vi "Add Injector.vi"(7 "Max Shots":T1(ring)=enum."1", 8 "error in (no error)":errorcluster, 9 "Stages":string[](array[string])=["Boost", "Battery", "Off"], 10 "Controls":T3[](array[typedef]) {"Data Type" format="%.0x"}, 11 "Item Ref":T2=18446744073709551615 format="%.0x") -> (0 "error out":errorcluster, 3 "Item Ref out":T2=18446744073709551615 format="%.0x")   [LabVIEW 2015, in "Fuel Injector Analysis Addon System Explorer.lvlib"]
uses:
  Fuel Injector Analysis Addon System Explorer.lvlib
  <vilib>/NI Veristand/Custom Device API/Custom Device Item Ref.ctl
  Shared/Types/Register.Info.ctl
  Shared/Types/FPGA Data Types.ctl
  FPGA/Injection Capture IP/Types/Injection.Global.Settings.ctl
  Shared/Constants.vi
  <vilib>/NI Veristand/Custom Device API/Set Item Property (Variant).vi
  <vilib>/NI Veristand/Custom Device Tools/Custom Device Utility Library/NI VeriStand - Search for Item by GUID.vi
  <vilib>/NI Veristand/Custom Device Tools/Custom Device Utility Library/NI VeriStand - Search for All Items by GUID.vi
  Shared/Fuel Injector Analysis Addon Shared.lvlib
  <vilib>/NI Veristand/Custom Device API/Custom Device API.lvlib
  <vilib>/NI Veristand/Custom Device Tools/Custom Device Utility Library/Custom Device Utility Library.lvlib
panel:
  in  "Tags":string
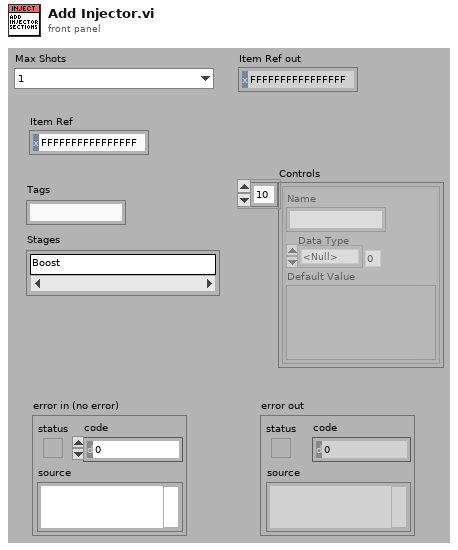
[diagram p1: front panel]
types:
  T1 = enum16{"0", "1", "2", "3", "4", "5", "6", "7", "8"}
  T2 = typedef "Custom Device API.lvlib/Custom Device Item Ref.ctl" = u64
  T3 = typedef "Fuel Injector Analysis Addon Shared.lvlib/Register.Info.ctl" = cluster{"Name":string, "Data Type":T4, "Default Value":variant}
  T4 = typedef "Fuel Injector Analysis Addon Shared.lvlib/FPGA Data Types.ctl" = enum8{"<Null>", "Injector.Core.Setting", "Injector.Global.Setting", "Injector.Mux.Setting", "Injector.Timing"}
  T5 = typedef "Injection.Global.Settings.ctl" = cluster{"Enable?":bool, "Initial Voltage Threshold":fxp<+/-,32,8>, "Event Dwell Limit":u16, "Voltage Gain":fxp<+/-,32,8>, "Current Gain":fxp<+/-,32,8>, "Filter Samples":u8, "Pretrigger Samples":u8}
  T6 = cluster{"Voltage Offset":fxp<+/-,32,8>, "Current Offset":fxp<+/-,32,8>}
  T7 = typedef "Fuel Injector Analysis Addon Shared.lvlib/Main Settings.ctl" = cluster{"RIO Device Address":string, "Local bitfile path":path, "RT bitfile path":path, "Number of injectors":u16, "Sample rate (S/s)":u32}
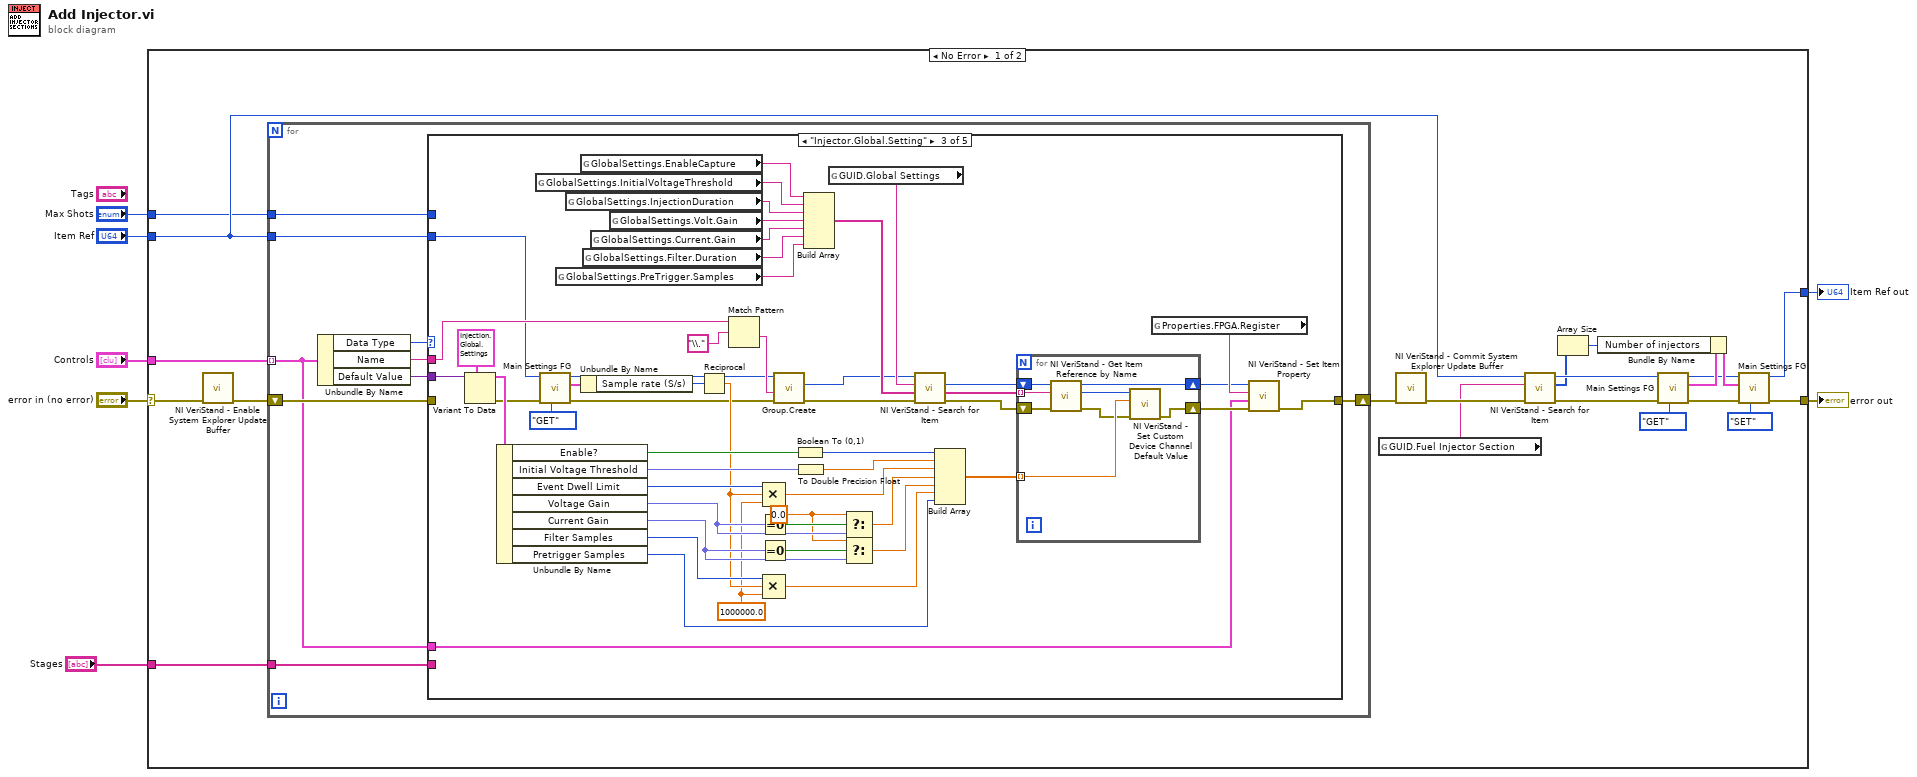
[diagram p0: block diagram]
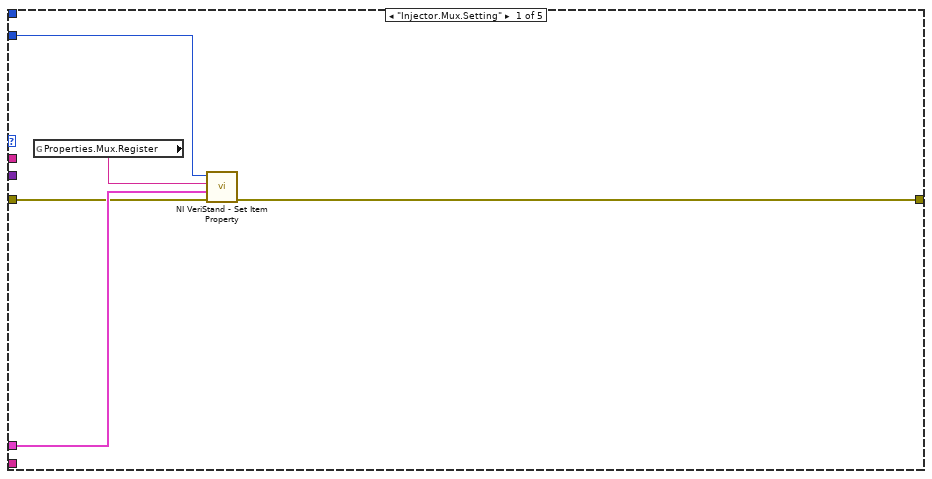
[diagram p2: hidden frame]
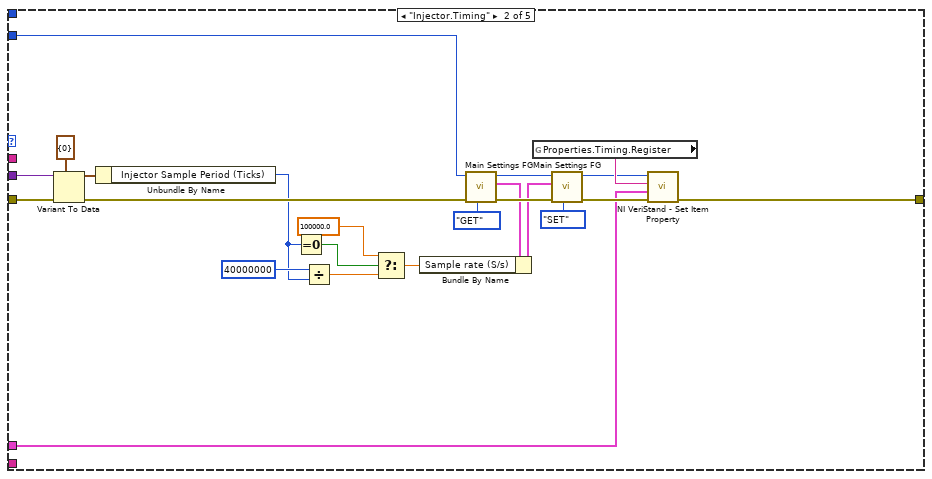
[diagram p3: hidden frame]
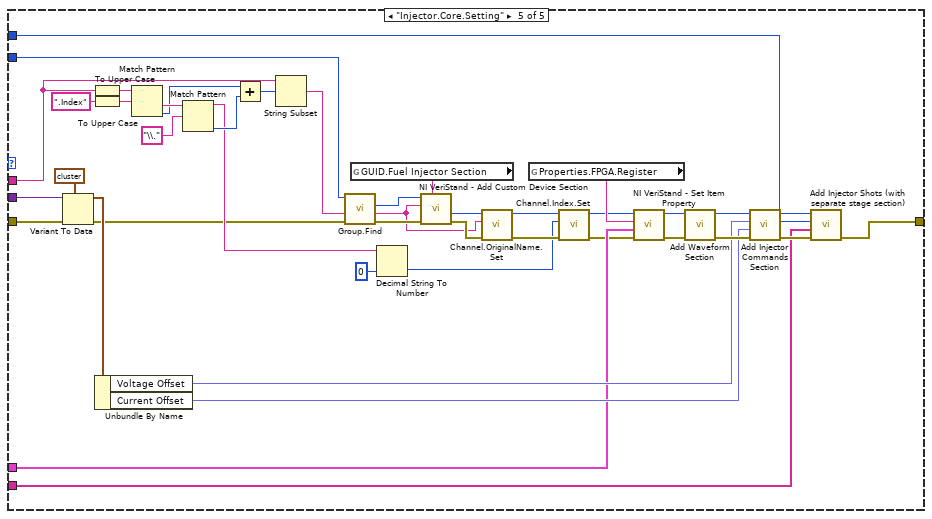
[diagram p5: hidden frame]
diagram:
  n1 = case shown="No Error" "error in (no error)" {
    selector: "error in (no error)" -> [w27 w168]
    tunnel: [w15 w168] -> w7
    tunnel: "Item Ref" -> [w20 w167]
    tunnel: "Controls" -> [w28 _]
    tunnel: [w14 w167] -> w3
    tunnel: "Stages" -> [w18 _]
    tunnel: "Max Shots" -> [w16 _]
    frame No Error {
      n2 = call <vilib>:"NI VeriStand - Enable System Explorer Update Buffer.vi"("error in (no error)"=w27) -> ("error out"=w19:errorcluster)  [unwired: 10 in]
      n3 = for {
        shift-right: [w36] -> w17
        shift-left: w19 -> [w37]
        tunnel: w28 -> [w34] mode=indexing
        tunnel: w18 -> [w31]
        tunnel: w16 -> [w30]
        tunnel: w20 -> [w29]
        n4 = Unbundle By Name(w34) -> ("Data Type"=w32:T4, "Name"=w33:string, "Default Value"=w35:variant)
        n5 = case shown="\"Injector.Global.Setting\"" w32 {
          tunnel: w37 -> [w39 w58 _ w124 w160]
          tunnel: [w38 w51 w99 w124 w161] -> w36
          tunnel: w29 -> [w40 w59 w70 _ w125]
          tunnel: w35 -> [_ w56 w115 _ w159]
          tunnel: w34 -> [w41 w48 w97 _ w151]
          tunnel: w33 -> [_ _ w72 _ w145]
          tunnel: w31 -> [_ _ _ _ w141]
          tunnel: w30 -> [_ _ _ _ w140]
          frame "Injector.Mux.Setting" {
            n6 = global read "Constants.vi" "Properties.Mux.Register"() -> (w42:string)
            n7 = call-poly <vilib>:"NI VeriStand - Set Item Property.vi"("error in (no error)"=w39, "Value"=w41, "Property Name"=w42, "Item Ref in"=w40) -> ("error out"=w38:errorcluster)  [unwired: 5 in, 2 out]
          }
          frame "Injector.Timing" {
            n8 = Variant To Data(error in=w58, type=cluster{"Injector Sample Period (Ticks)":u32} {"Injector Sample Period (Ticks)"=0} ("Injector.Timing"), Variant=w56) -> (data=w49:cluster{"Injector Sample Period (Ticks)":u32}, error out=w57:errorcluster)
            n9 = Unbundle By Name(w49) -> ("Injector Sample Period (Ticks)"=w47:u32)
            n10 = Equal To 0?(x=w47) -> (x = 0?=w46:bool)
            n11 = Divide(x=u32 40000000, y=w47) -> (x/y=w44:dbl)
            n12 = Select(t=100000.0, s=w46, f=w44) -> (s? t:f=w43:dbl)
            n13 = call "Main Settings FG.vi"("Action"=enum8{"GET", "SET"}."GET", "error in (no error)"=w57, "Item Ref"=w59) -> ("error out"=w65:errorcluster, "Main Settings out"=w64:T7, "Item Ref out"=w61:T2)  [unwired: 6 in]
            n14 = Bundle By Name(cluster=w64, "Sample rate (S/s)"=w43) -> (w63:T7)
            n15 = global read "Constants.vi" "Properties.Timing.Register"() -> (w53:string)
            n16 = call "Main Settings FG.vi"("Action"=enum8{"GET", "SET"}."SET", "error in (no error)"=w65, "Main Settings"=w63, "Item Ref"=w61) -> ("error out"=w52:errorcluster, "Item Ref out"=w50:T2)  [unwired: 5 in, 1 out]
            n17 = call-poly <vilib>:"NI VeriStand - Set Item Property.vi"("error in (no error)"=w52, "Value"=w48, "Property Name"=w53, "Item Ref in"=w50) -> ("error out"=w51:errorcluster)  [unwired: 5 in, 2 out]
          }
          frame "Injector.Global.Setting" {
            w75 = 1000000.0 ("value")
            w83 = 0.0 ("x*y")
            n18 = Variant To Data(type=T5 {"Enable?"=FALSE, "Initial Voltage Threshold"=0.0, "Event Dwell Limit"=0, "Voltage Gain"=0.0, "Current Gain"=1.0, "Filter Samples"=5, "Pretrigger Samples"=5} ("InjectorAnalysis.Settings"), Variant=w115) -> (data=w114:T5, error out=w104:errorcluster)  [unwired: 1 in]
            n19 = Unbundle By Name(w114) -> ("Enable?"=w108:bool, "Initial Voltage Threshold"=w109:fxp<+/-,32,8>, "Event Dwell Limit"=w102:u16, "Voltage Gain"=w96:fxp<+/-,32,8>, "Current Gain"=w95:fxp<+/-,32,8>, "Filter Samples"=w78:u8, "Pretrigger Samples"=w74:u8)
            n20 = global read "Constants.vi" "GlobalSettings.InitialVoltageThreshold"() -> (w81:string)
            n21 = call "Main Settings FG.vi"("Action"=enum8{"GET", "SET"}."GET", "error in (no error)"=w104, "Item Ref"=w70) -> ("error out"=w67:errorcluster, "Main Settings out"=w106:T7, "Item Ref out"=w68:T2)  [unwired: 6 in]
            n22 = global read "Constants.vi" "GlobalSettings.PreTrigger.Samples"() -> (w79:string)
            n23 = global read "Constants.vi" "GlobalSettings.InjectionDuration"() -> (w92:string)
            n24 = global read "Constants.vi" "GlobalSettings.EnableCapture"() -> (w93:string)
            n25 = Unbundle By Name(w106) -> ("Sample rate (S/s)"=w103:u32)
            n26 = global read "Constants.vi" "GlobalSettings.Filter.Duration"() -> (w80:string)
            n27 = global read "Constants.vi" "GlobalSettings.Current.Gain"() -> (w90:string)
            n28 = global read "Constants.vi" "GlobalSettings.Volt.Gain"() -> (w91:string)
            n29 = Reciprocal(x=w103) -> (1/x=w77:dbl)
            n30 = Match Pattern(string=w72, regular expression="\\.") -> (after substring=w71:string)  [unwired: 1 in, 3 out]
            n31 = Equal To 0?(x=w96) -> (x = 0?=w87:bool)
            n32 = Equal To 0?(x=w95) -> (x = 0?=w84:bool)
            n33 = Compound Arithmetic op=MULTIPLY(w102, w77, w75) -> (w85:dbl)
            n34 = Compound Arithmetic op=MULTIPLY(w78, w77, w75) -> (w76:dbl)
            n35 = call "Group.Create.vi"("error in (no error)"=w67, "Name"=w71, "Parent"=w68) -> ("error out"=w66:errorcluster, "Child"=w69:T2)  [unwired: 6 in, 1 out]
            n36 = Boolean To (0,1)(Boolean=w108) -> (0, 1=w89:i16)
            n37 = To Double Precision Float(number=w109) -> (double precision float=w88:dbl)
            n38 = Build Array(w93, w81, w92, w91, w90, w80, w79) -> (w111:string[])
            n39 = global read "Constants.vi" "GUID.Global Settings"() -> (w112:string)
            n40 = Select(t=w83, s=w87, f=w96) -> (s? t:f=w86:dbl)
            n41 = Select(t=w83, s=w84, f=w95) -> (s? t:f=w82:dbl)
            n42 = call-poly <vilib>:"NI VeriStand - Search for Item.vi"("error in"=w66, "Item GUID"=w112, "Section Ref in"=w69) -> ("error out"=w110:errorcluster, "Item Ref"=w94:T2)  [unwired: 5 in, 2 out]
            n43 = Build Array(w89, w88, w85, w86, w82, w76, w74) -> (w107:dbl[])
            n44 = for {
              tunnel: w111 -> [w120] mode=indexing
              shift-right: [w123] -> w100
              shift-left: w110 -> [w119]
              tunnel: w107 -> [w122] mode=indexing
              shift-right: [w117] -> w98
              shift-left: w94 -> [w121]
              n45 = call <vilib>:"NI VeriStand - Get Item Reference by Name.vi"("error in (no error)"=w119, "Item Name"=w120, "Parent Ref in"=w121) -> ("error out"=w118:errorcluster, "Item Ref"=w116:T2, "Parent Ref out"=w117:T2)  [unwired: 5 in, 1 out]
              n46 = call <vilib>:"NI VeriStand - Set Custom Device Channel Default Value.vi"("error in (no error)"=w118, "Default Value"=w122, "Channel Ref in"=w116) -> ("error out"=w123:errorcluster)  [unwired: 7 in, 1 out]
            }
            n47 = global read "Constants.vi" "Properties.FPGA.Register"() -> (w101:string)
            n48 = call-poly <vilib>:"NI VeriStand - Set Item Property.vi"("error in (no error)"=w100, "Value"=w97, "Property Name"=w101, "Item Ref in"=w98) -> ("error out"=w99:errorcluster)  [unwired: 5 in, 2 out]
          }
          frame "<Null>", Default {
          }
          frame "Injector.Core.Setting" {
            n49 = Variant To Data(error in=w160, type=T6 {"Voltage Offset"=0.0, "Current Offset"=0.0} ("Injector.Core.Settings Ch5"), Variant=w159) -> (data=w157:T6, error out=w130:errorcluster)
            n50 = To Upper Case(1:w145) -> (0:w149:string)
            n51 = To Upper Case(1:".Index" ("regular expression")) -> (0:w148:string)
            n52 = Unbundle By Name(w157) -> ("Voltage Offset"=w156:fxp<+/-,32,8>, "Current Offset"=w155:fxp<+/-,32,8>)
            n53 = Match Pattern(string=w149, regular expression=w148) -> (after substring=w147:string, offset past match=w144:i32)  [unwired: 1 in, 2 out]
            n54 = Match Pattern(string=w147, regular expression="\\.") -> (before substring=w137:string, offset past match=w143:i32)  [unwired: 1 in, 2 out]
            n55 = Add(x=w144, y=w143) -> (x+y=w142:i32)
            n56 = String Subset(string=w145, offset (0)=w142) -> (substring=w126:string)  [unwired: 1 in]
            n57 = call "Group.Find.vi"("error in (no error)"=w130, "Name"=w126, "Parent"=w125) -> ("error out"=w129:errorcluster, "Child Name"=w128:string, "Child"=w127:T2)  [unwired: 5 in, 1 out]
            n58 = global read "Constants.vi" "GUID.Fuel Injector Section"() -> (w164:string)
            n59 = Decimal String To Number(string=w137, default (0L)=u16 0 ("default (0 I32)")) -> (number=w131:u16)  [unwired: 1 in, 1 out]
            n60 = call <vilib>:"NI VeriStand - Add Custom Device Section.vi"("GUID (Default Section)"=w164, "error in (no error)"=w129, "Section Name"=w128, "Parent Ref in"=w127) -> ("error out"=w138:errorcluster, "Section Ptr"=w139:T2)  [unwired: 4 in, 2 out]
            n61 = call "Channel.OriginalName.Set.vi"("error in (no error)"=w138, "Constants.Channel Name"=w128, "Ref"=w139) -> ("error out"=w134:errorcluster, "Ref out"=w135:T2)  [unwired: 7 in]
            n62 = global read "Constants.vi" "Properties.FPGA.Register"() -> (w152:string)
            n63 = call "Channel.Index.Set.vi"("error in (no error)"=w134, "Constants.Index"=w131, "Ref"=w135) -> ("error out"=w132:errorcluster, "Ref out"=w133:T2)  [unwired: 7 in]
            n64 = call-poly <vilib>:"NI VeriStand - Set Item Property.vi"("error in (no error)"=w132, "Value"=w151, "Property Name"=w152, "Item Ref in"=w133) -> ("error out"=w154:errorcluster, "Item Ref out"=w153:T2)  [unwired: 5 in, 1 out]
            n65 = call "Add Waveform Section.vi"("error in (no error)"=w154, "Section Ptr"=w153) -> ("error out"=w166:errorcluster, "Injector Section ptr"=w165:T2)  [unwired: 8 in]
            n66 = call "Add Injector Commands Section.vi"("error in (no error)"=w166, "Default Current Offset"=w155, "Default Volt Offset"=w156, "Injector Section ptr"=w165) -> ("error out"=w162:errorcluster, "Parent Ref out"=w163:T2)  [unwired: 6 in]
            n67 = call "Add Injector Shots (with separate stage section).vi"("error in (no error)"=w162, "Stage Names"=w141, "# shots to add"=w140, "Injector Section Ref in"=w163) -> ("error out"=w161:errorcluster)  [unwired: 7 in]
          }
        }
      }
      n68 = global read "Constants.vi" "GUID.Fuel Injector Section"() -> (w10:string)
      n69 = call <vilib>:"NI VeriStand - Commit System Explorer Update Buffer.vi"("error in (no error)"=w17) -> ("error out"=w13:errorcluster)  [unwired: 10 in]
      n70 = call-poly <vilib>:"NI VeriStand - Search for Item.vi"("error in"=w13, "Item GUID"=w10, "Section Ref in"=w20) -> ("error out"=w12:errorcluster, "Item Refs"=w9:T2[], "Section Ref out"=w11:T2)  [unwired: 5 in, 1 out]
      n71 = Array Size(array=w9) -> (size(s)=w8:i32)
      n72 = call "Main Settings FG.vi"("Action"=enum8{"GET", "SET"}."GET", "error in (no error)"=w12, "Item Ref"=w11) -> ("error out"=w26:errorcluster, "Main Settings out"=w25:T7, "Item Ref out"=w22:T2)  [unwired: 6 in]
      n73 = Bundle By Name(cluster=w25, "Number of injectors"=w8) -> (w24:T7)
      n74 = call "Main Settings FG.vi"("Action"=enum8{"GET", "SET"}."SET", "error in (no error)"=w26, "Main Settings"=w24, "Item Ref"=w22) -> ("error out"=w15:errorcluster, "Item Ref out"=w14:T2)  [unwired: 5 in, 1 out]
    }
    frame Error {
    }
  }
  "error out" <- w7
  "Item Ref out" <- w3
